vi "predict state.vi"(10 "x_k-1|k-1":T1, 11 "F_k":T1) -> (3 "x_k|k-1":T1)   [LabVIEW 2016]
uses:
  <vilib>/Analysis/Matrix/Datatypes/RealMatrix.ctl
  <vilib>/Analysis/baseanly.llb/Real A x B.vi
  <vilib>/Analysis/NI_AALBase.lvlib
  <vilib>/Analysis/Matrix/NI_Matrix.lvlib
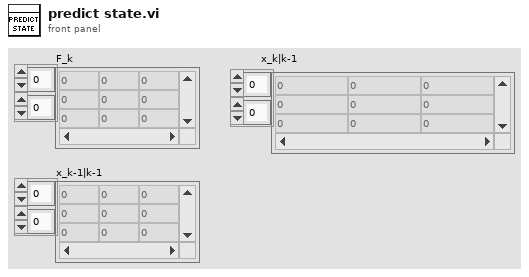
[diagram p1: front panel]
types:
  T1 = typedef "NI_Matrix.lvlib/RealMatrix.ctl" = dbl[][]
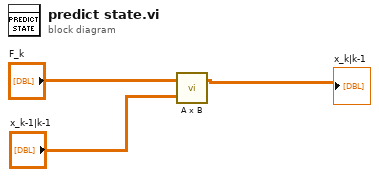
[diagram p0: block diagram]
diagram:
  n1 = call-poly <vilib>:"A x B.vi"("B"="x_k-1|k-1", "A"="F_k") -> ("A x B"=→"x_k|k-1":T1)  [unwired: 1 out]
